vi "graphs.vi"() -> ()   [LabVIEW 2018]
uses:
  <vilib>/express/express arith-compare/Formula/XNode/ExpressFormulaBlockNode.xnode
panel:
  in  "Tab Control":enum32{"Page 1", "Page 2", "Page 3", "Page 4"}(tab)
  out "Sine":dynamicdata(graph)
  out "Waveform Chart":dbl(graph)
  in  "Numeric 3":i32
  in  "Reset Signal":bool
  in  "Offset":dbl
  in  "Phase":dbl
  in  "Frequency":dbl=10.1
  in  "Amplitude":dbl=1.0
  in  "X1":dbl
  in  "Numeric 2":dbl
  out "Numeric":dbl
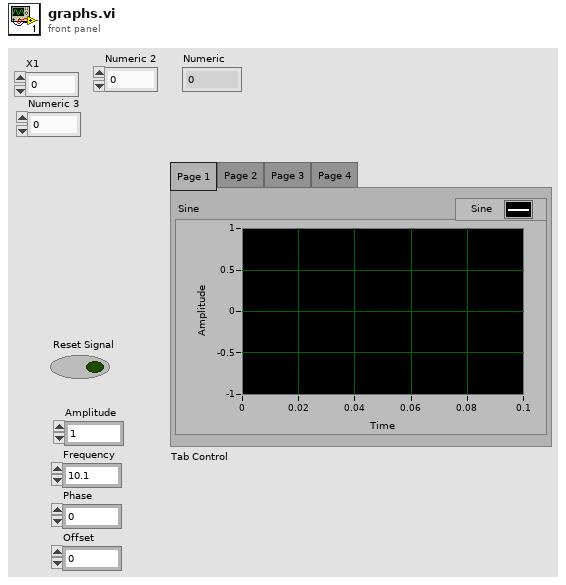
[diagram p1: front panel]
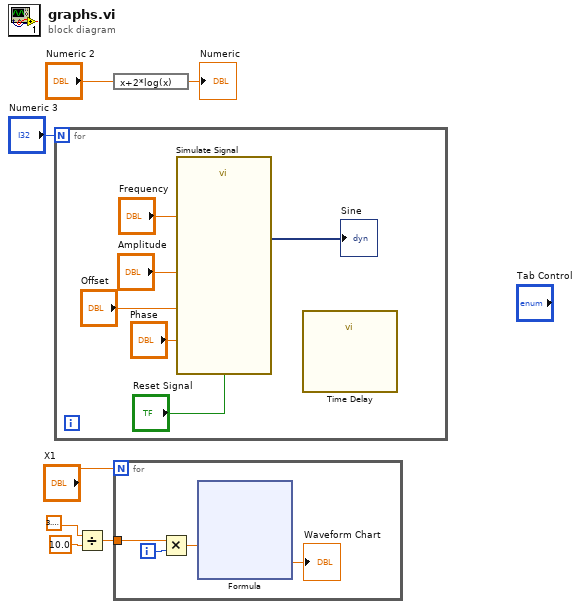
[diagram p0: block diagram]
diagram:
  n1 = for {
    N: "Numeric 3" -> [_]
    n2 = call "Simulate Signal"("Offset"="Offset", "Reset Signal"="Reset Signal", "Frequency"="Frequency", "Amplitude"="Amplitude", "Phase"="Phase") -> ("Sine"=→"Sine":dynamicdata)  [unwired: 9 in, 1 out]
    n3 = call "Time Delay"() -> ()  [unwired: 11 in, 1 out]
  }
  n4 = Divide(x=3.141592653589793, y=10.0) -> (x/y=w2:dbl)
  n5 = expression code="x+2*log(x)"("Numeric 2") -> (→"Numeric":dbl)
  n6 = for {
    N: "X1" -> [_]
    tunnel: w2 -> [w16]
    i -> [w17]
    n7 = Multiply(x=w16, y=w17) -> (x*y=w15:dbl)
    n8 = xnode "Formula"("X1"=w15) -> ("Result"=→"Waveform Chart":dbl)  [unwired: 1 in, 1 out]
  }
